vi "Get All Paths.vi"(11 "Parsed Results Data (by VI)":T1[](array[typedef])) -> (3 "Array":path[](array[path]))   [LabVIEW 2019]
uses:
  <vilib>/addons/analyzer/_vianresshared.llb/VIAnRes Parsed Results Data (by VI).ctl
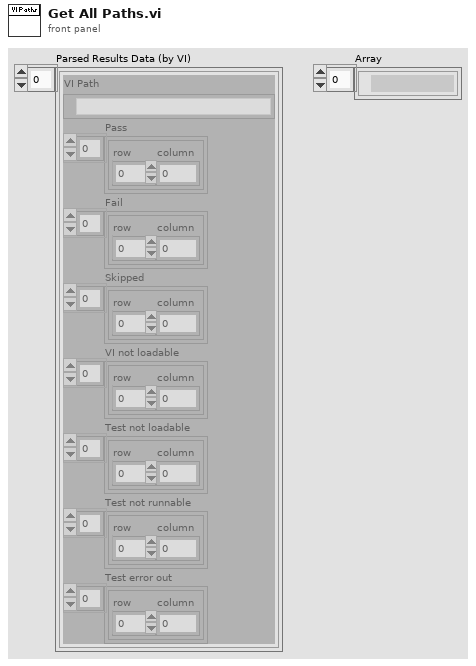
[diagram p1: front panel]
types:
  T1 = typedef "VIAnRes Parsed Results Data (by VI).ctl" = cluster{"VI Path":path, "Pass":cluster{"row":i32, "column":i32}[], "Fail":cluster{"row":i32, "column":i32}[], "Skipped":cluster{"row":i32, "column":i32}[], "VI not loadable":cluster{"row":i32, "column":i32}[], "Test not loadable":cluster{"row":i32, "column":i32}[], "Test not runnable":cluster{"row":i32, "column":i32}[], "Test error out":cluster{"row":i32, "column":i32}[]}
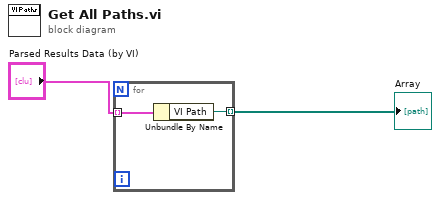
[diagram p0: block diagram]
diagram:
  n1 = for {
    tunnel: "Parsed Results Data (by VI)" -> [w4] mode=indexing
    tunnel: [w3] -> w1 mode=indexing
    n2 = Unbundle By Name(w4) -> ("VI Path"=w3:path)
  }
  "Array" <- w1
